vi "WS1050_36 DUT CV Curve SData Ver1.3.vi"(0 "TMN DC\\CAP Data Log File Path":path=path "C:/temp", 1 "Lot#":string="WS1050", 4 "Wafer#":string="T7", 5 "File Name":string="Test Data", 7 "error in":errorcluster, 8 "TP/Comment":T1={"Test Program"="Multi Socket", "Comment"="HD_Cycling", "DVA"="", "EFUSE CAL"="", "CP HD/CYC"="", "VDD"="", "Duty Cycle"="", "V_Test(V)"="", "V_VPI(V)"="", "Freq(Hz)"="", "Board#"=""}, 9 "EFuse":string[](array[string])=["NC", "NC", "NC", "NC", "NC", "NC", "NC", "NC", "NC", "NC", "NC", "NC", "NC", "NC", "NC", "NC", "NC", "NC", "NC", "NC", "NC", "NC", "NC", "NC", "NC", "NC", "NC", "NC", "NC", "NC", "NC", "NC", "NC", "NC", "NC", "NC"], 10 "Data Output C3":string[][](table), 11 "Temperature":string="WS1033", 13 "VPI C3":string[][](array[string]), 14 "Data Output C1":string[][](table), 15 "VPI C2":string[][](array[string]), 16 "SN":string[](array[string])=["1", "2", "3", "4", "5", "6", "7", "8", "9", "10", "11", "12", "13", "14", "15", "16", "17", "18", "19", "20", "21", "22", "23", "24", "25", "26", "27", "28", "29", "30", "31", "32", "33", "34", "35", "36"], 17 "R/W Status":string[](array[string])=["PASS", "PASS", "PASS", "PASS", "PASS", "PASS", "PASS", "PASS", "PASS", "PASS", "PASS", "PASS", "PASS", "PASS", "PASS", "PASS", "PASS", "PASS", "PASS", "PASS", "PASS", "PASS", "PASS", "PASS", "PASS", "PASS", "PASS", "PASS", "PASS", "PASS", "PASS", "PASS", "PASS", "PASS", "PASS", "PASS"], 18 "Cap Header":string[](array[string]), 20 "HD/Cycles Completed":string="Test Data", 21 "Data Output C2":string[][](table), 24 "Current":string[](array[string]), 25 "VPI C1":string[][](array[string])) -> (27 "error out":errorcluster)   [LabVIEW 2012]
doc: "WS1050, 36DUT CP Sweep Save Data"
panel:
  in  "Bin":string[](array[string])=["NC", "NC", "NC", "NC", "NC", "NC", "NC", "NC", "NC", "NC", "NC", "NC", "NC", "NC", "NC", "NC", "NC", "NC", "NC", "NC", "NC", "NC", "NC", "NC", "NC", "NC", "NC", "NC", "NC", "NC", "NC", "NC", "NC", "NC", "NC", "NC"]
  # "*********** Do Not Remove ***********\nCompany:  WiSpry Inc\n20 Fairbanks Ste 198 Irvine CA 92618\n\nAuthor:  Andy V Tran\nCreated:  07/07/2016\nLabVIEW 2012 Suite\nTP:  Multi-Socket Save Data ver1.3\n*****************************************"
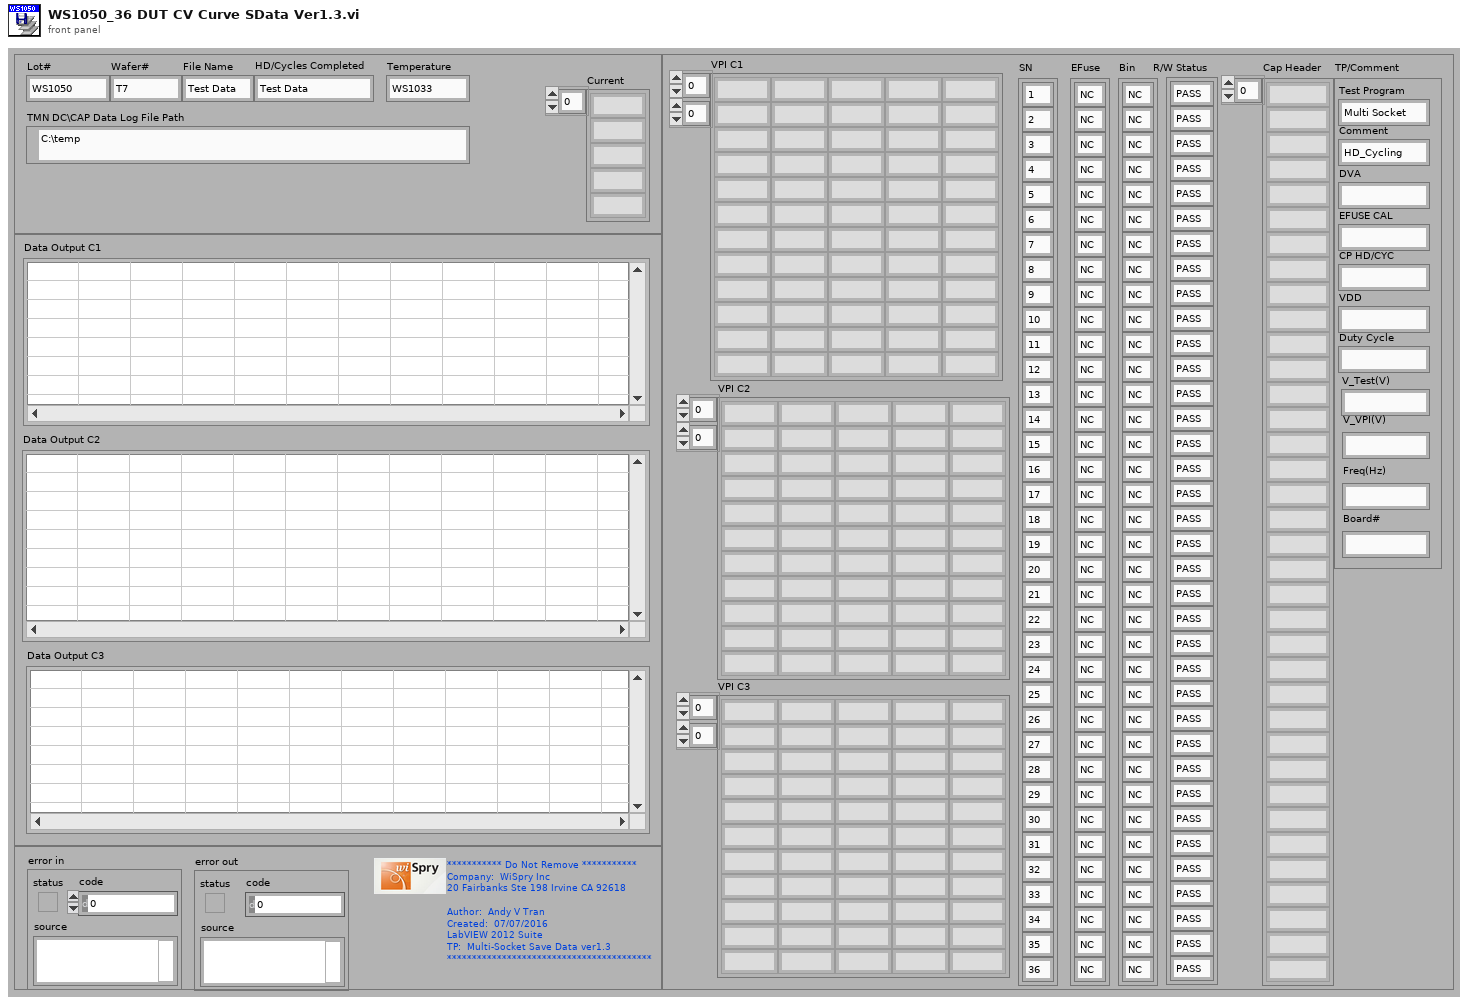
[diagram p1: front panel]
types:
  T1 = cluster{"Test Program":string, "Comment":string, "DVA":string, "EFUSE CAL":string, "CP HD/CYC":string, "VDD":string, "Duty Cycle":string, "V_Test(V)":string, "V_VPI(V)":string, "Freq(Hz)":string, "Board#":string}
  T2 = enum16{"open", "replace", "create", "open or create", "replace or create", "replace or create with confirmation"}
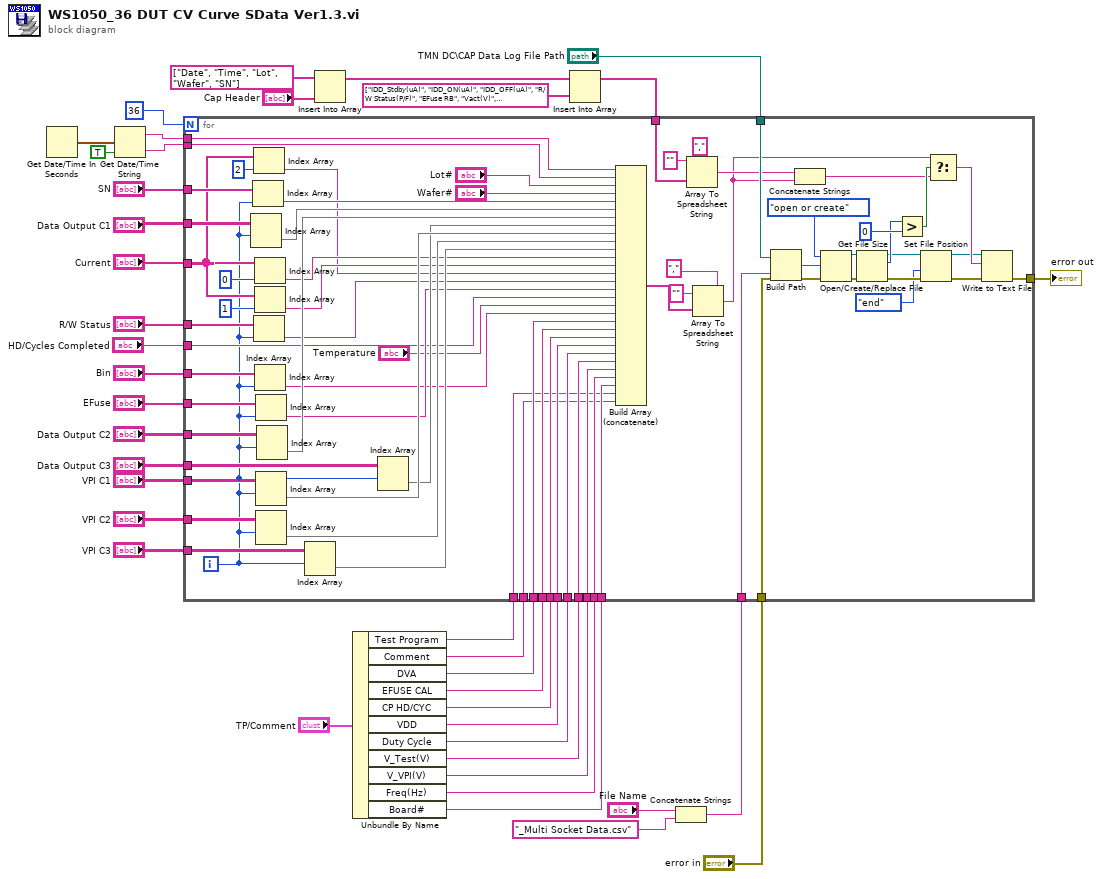
[diagram p0: block diagram]
diagram:
  n1 = Get Date/Time In Seconds() -> (seconds since 1Jan1904=w19:timestamp)
  n2 = Get Date/Time String(seconds (now)=w19, want seconds? (F)=TRUE) -> (date string=w27:string, time string=w28:string)  [unwired: 1 in]
  n3 = Insert Into Array(array=string[] ["Date", "Time", "Lot", "Wafer", "SN"], new element="Cap Header") -> (w12:string[])  [unwired: 1 in]
  n4 = Unbundle By Name("TP/Comment") -> ("Test Program"=w32:string, "Comment"=w31:string, "DVA"=w11:string, "EFUSE CAL"=w10:string, "CP HD/CYC"=w9:string, "VDD"=w8:string, "Duty Cycle"=w7:string, "V_Test(V)"=w6:string, "V_VPI(V)"=w5:string, "Freq(Hz)"=w3:string, "Board#"=w2:string)
  n5 = Insert Into Array(array=w12, new element=string[] ["IDD_Stdby(uA)", "IDD_ON(uA)", "IDD_OFF(uA)", "R/W Status(P/F)", "EFuse RB", "Vact(V)", "Temperature", "Bin", "DVA ON/OFF", "CAL ON/OFF", "CP_Sweep(V)", "VDD", "Duty Cycle(%)", "V_Test(V)", "V_VPI(V)", "Freq(Hz)", "Board", "Test Program", "Comment"]) -> (w13:string[])  [unwired: 1 in]
  n6 = Concatenate Strings("File Name", "_Multi Socket Data.csv" ("string")) -> (w35:string)
  n7 = for {
    N: 36 -> [_]
    tunnel: "TMN DC\\CAP Data Log File Path" -> [w111]
    tunnel: w13 -> [w110]
    tunnel: "error in" -> [w74]
    tunnel: w35 -> [w109]
    tunnel: [w87] -> w34
    tunnel: "SN" -> [w86]
    tunnel: "Current" -> [w78]
    tunnel: w32 -> [w43]
    tunnel: w31 -> [w42]
    tunnel: "Bin" -> [w85]
    tunnel: "R/W Status" -> [w84]
    tunnel: w28 -> [w64]
    tunnel: w27 -> [w63]
    tunnel: "Data Output C1" -> [w83]
    tunnel: "Data Output C2" -> [w82]
    tunnel: "VPI C1" -> [w77]
    tunnel: "VPI C2" -> [w76]
    tunnel: "EFuse" -> [w75]
    tunnel: "VPI C3" -> [w73]
    tunnel: "Data Output C3" -> [w72]
    tunnel: w11 -> [w52]
    tunnel: w10 -> [w51]
    tunnel: w9 -> [w50]
    tunnel: w8 -> [w49]
    tunnel: w7 -> [w48]
    tunnel: w6 -> [w47]
    tunnel: w5 -> [w46]
    tunnel: "HD/Cycles Completed" -> [w55]
    tunnel: w3 -> [w45]
    tunnel: w2 -> [w44]
    i -> [w41]
    n8 = Index Array(array=w83, index (row)=w41) -> (element=w66:string[])  [unwired: 1 in]
    n9 = Index Array(array=w86, index=w41) -> (element=w65:string)
    n10 = Index Array(array=w78, index=2) -> (element=w58:string)
    n11 = Index Array(array=w84, index=w41) -> (element=w57:string)
    n12 = Index Array(array=w78, index=0) -> (element=w60:string)
    n13 = Index Array(array=w78, index=1) -> (element=w59:string)
    n14 = Index Array(array=w85, index=w41) -> (element=w53:string)
    n15 = Index Array(array=w75, index=w41) -> (element=w56:string)
    n16 = Index Array(array=w77, index (row)=w41) -> (element=w69:string[])  [unwired: 1 in]
    n17 = Index Array(array=w76, index (row)=w41) -> (element=w70:string[])  [unwired: 1 in]
    n18 = Index Array(array=w82, index (row)=w41) -> (element=w67:string[])  [unwired: 1 in]
    n19 = Index Array(array=w73, index (row)=w41) -> (element=w71:string[])  [unwired: 1 in]
    n20 = Index Array(array=w72, index (row)=w41) -> (element=w68:string[])  [unwired: 1 in]
    n21 = Build Array (concatenate)(w63, w64, "Lot#", "Wafer#", w65, w66, w67, w68, w69, w70, w71, w60, w59, w58, w57, w56, w55, "Temperature", w53, w52, w51, w50, w49, w48, w47, w46, w45, w44, w43, w42) -> (w88:string[])
    n22 = Array To Spreadsheet String(delimiter (Tab)=",", array=w110, 3:"" ("format string")) -> (spreadsheet string=w91:string)
    n23 = Array To Spreadsheet String(delimiter (Tab)=",", array=w88, 3:"" ("format string")) -> (spreadsheet string=w89:string)
    n24 = Build Path(base path=w111, name or relative path=w109) -> (appended path=w103:path)
    n25 = Concatenate Strings(w91, w89) -> (w90:string)
    n26 = Open/Create/Replace File(file path (use dialog)=w103, error in=w74, operation (0:open)=T2."open or create") -> (refnum out=w101:refnum<file>, error out=w104:errorcluster)  [unwired: 4 out]
    n27 = Get File Size(file=w101, error in=w104) -> (refnum out=w96:refnum<file>, size (in bytes)=w100:i64, 0:w98:errorcluster)
    n28 = Greater?(x=w100, y=i64 0) -> (0:w105:bool)
    n29 = Set File Position(refnum=w96, from (0:start)=enum16{"start", "end", "current"}."end", error in=w98) -> (refnum out=w95:refnum<file>, error out=w97:errorcluster)  [unwired: 1 out]
    n30 = Select(t=w89, s=w105, f=w90) -> (s? t:f=w102:string)
    n31 = Write to Text File(file (use dialog)=w95, text=w102, error in=w97) -> (error out=w87:errorcluster)  [unwired: 3 out]
  }
  "error out" <- w34
